vi "Build Target.vi"(8 "error in (no error)":errorcluster, 10 "Skip Core":bool, 11 "Target":T1) -> (0 "error out":errorcluster)   [LabVIEW 2017]
uses:
  Target Type.ctl
  Constants.vi
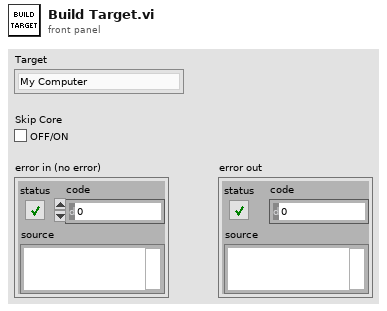
[diagram p1: front panel]
types:
  T1 = typedef "Target Type.ctl" = enum16{"My Computer", "Pharlap"}
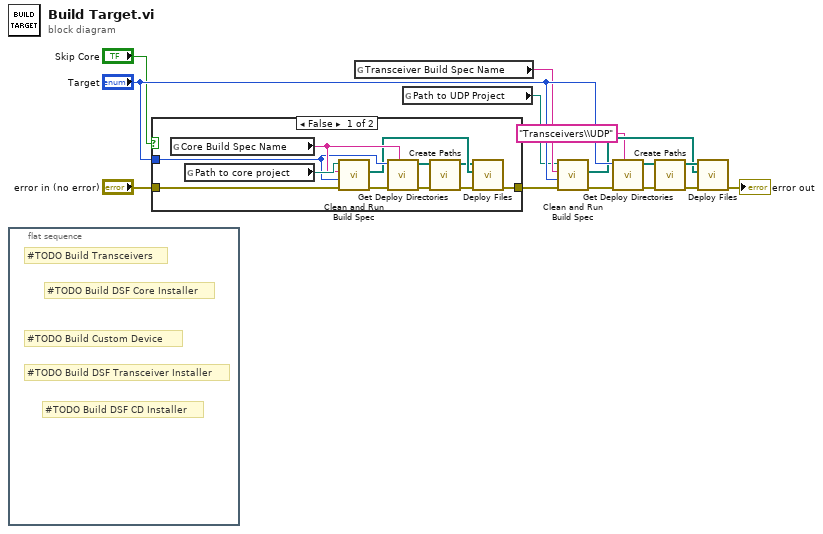
[diagram p0: block diagram]
diagram:
  n1 = flat-sequence {
    frame #0 {
      # "#TODO Build DSF CD Installer"
      # "#TODO Build DSF Transceiver Installer"
      # "#TODO Build DSF Core Installer"
      # "#TODO Build Custom Device"
      # "#TODO Build Transceivers"
    }
  }
  n2 = case shown="False" "Skip Core" {
    tunnel: "error in (no error)" -> [w20 w26]
    tunnel: "Target" -> [w19 _]
    tunnel: [w15 w26] -> w11
    frame False {
      n3 = global read "Constants.vi" "Core Build Spec Name"() -> (w21:string)
      n4 = global read "Constants.vi" "Path to core project"() -> (w25:path)
      n5 = call "Clean and Run Build Spec.vi"("error in (no error)"=w20, "Target"=w19, "Name of build specification"=w21, "Path to project"=w25) -> ("error out"=w23:errorcluster, "Generated files"=w17:path[])  [unwired: 6 in]
      n6 = call "Get Deploy Directories.vi"("Subdirectory"=w21, "error in (no error)"=w23, "Target"=w19) -> ("error out"=w22:errorcluster, "Directories to Deploy To"=w24:path[])  [unwired: 7 in]
      n7 = call "Create Paths.vi"("error in (no error)"=w22, "Paths"=w24) -> ("error out"=w18:errorcluster, "Paths out"=w16:path[])  [unwired: 8 in]
      n8 = call "Deploy Files.vi"("error in (no error)"=w18, "Generated files"=w17, "Paths in"=w16) -> ("error out"=w15:errorcluster)  [unwired: 8 in]
    }
    frame True {
    }
  }
  n9 = global read "Constants.vi" "Transceiver Build Spec Name"() -> (w12:string)
  n10 = global read "Constants.vi" "Path to UDP Project"() -> (w9:path)
  n11 = call "Clean and Run Build Spec.vi"("error in (no error)"=w11, "Target"="Target", "Name of build specification"=w12, "Path to project"=w9) -> ("error out"=w4:errorcluster, "Generated files"=w3:path[])  [unwired: 6 in]
  n12 = call "Get Deploy Directories.vi"("Subdirectory"="Transceivers\\UDP", "error in (no error)"=w4, "Target"="Target") -> ("error out"=w7:errorcluster, "Directories to Deploy To"=w8:path[])  [unwired: 7 in]
  n13 = call "Create Paths.vi"("error in (no error)"=w7, "Paths"=w8) -> ("error out"=w5:errorcluster, "Paths out"=w6:path[])  [unwired: 8 in]
  n14 = call "Deploy Files.vi"("error in (no error)"=w5, "Generated files"=w3, "Paths in"=w6) -> ("error out"=→"error out":errorcluster)  [unwired: 8 in]
